vi "Stop Core.vi"(10 "final error code":i32, 11 "NI_DAQmx(Linear) in":refnum<class "NI_DAQmx(Linear).lvclass">) -> (3 "NI_DAQmx(Linear) out":refnum<class "NI_DAQmx(Linear).lvclass">)   [LabVIEW 2025, in "NI_DAQmx(Linear).lvclass"]
doc: "<p>(<strong>Filename</strong>: <span class=\"dnl\">Actor Framework.lvlib:Actor.lvclass:Stop Core.vi</span>)</p>\n<p>Defines what the actor does before it stops. Use the <strong>final error code</strong> input to determine whether the actor shut down in response to an error.</p>\n<p>By default, this method passes the Stop message along to all <a href=\"nihelplauncher://docs/csh?context=lvcore_lvcomm_af_launch_nested_actor\">auto-stop nested actors</a>. A descendant class may override this method to define additional behavior, such as shutting down any processes the actor initiated in its override of the <a href=\"nihelplauncher://docs/csh?context=lvcore_lvcomm_af_actor_core\">Actor Core</a> method.</p>"
uses:
  NI_DAQmx(Linear).lvclass
  NI_DAQmx(Linear).lvclass/NI_DAQmx(Linear).ctl
  Read task.vi
  DAQ_Abstr/Task_Type/Linear_Task/Linear_Task/Linear_Task.lvclass
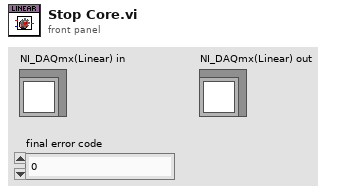
[diagram p1: front panel]
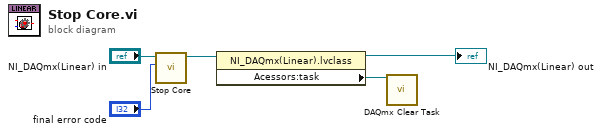
[diagram p0: block diagram]
diagram:
  n1 = call-parent "Stop Core.vi"("final error code"="final error code", "Task_Abstr in"="NI_DAQmx(Linear) in") -> ("Task_Abstr out"=w2:refnum<class "NI_DAQmx(Linear).lvclass">)  [unwired: 9 in]
  n2 = property class="NI_DAQmx(Linear).lvclass"(reference=w2) -> (reference out=→"NI_DAQmx(Linear) out":refnum<class "NI_DAQmx(Linear).lvclass">, "Acessors:task"=w3:refnum<k21>)  [unwired: 1 in, 1 out]
  n3 = call <vilib>:"DAQmx Clear Task.vi"("task in"=w3) -> ()  [unwired: 14 in, 1 out]
